vi "OutputDebugString.vi"(6 "Force Log":bool, 8 "error in (log if error)":errorcluster, 11 "log entry string":string) -> (0 "error out":errorcluster, 1 "ms value":u32, 2 "date/time string":string, 3 "data logged":string)   [LabVIEW 2020]
uses:
  Kernel32.dll
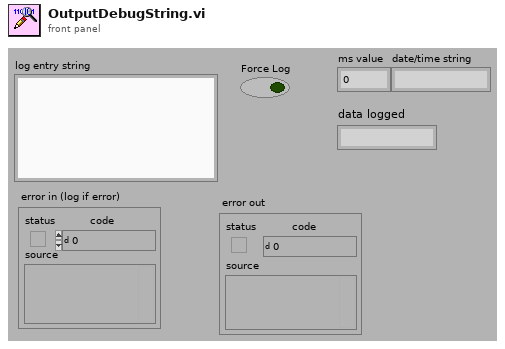
[diagram p1: front panel]
types:
  T1 = enum16{"open", "replace", "create", "open or create", "replace or create", "replace or create with confirmation"}
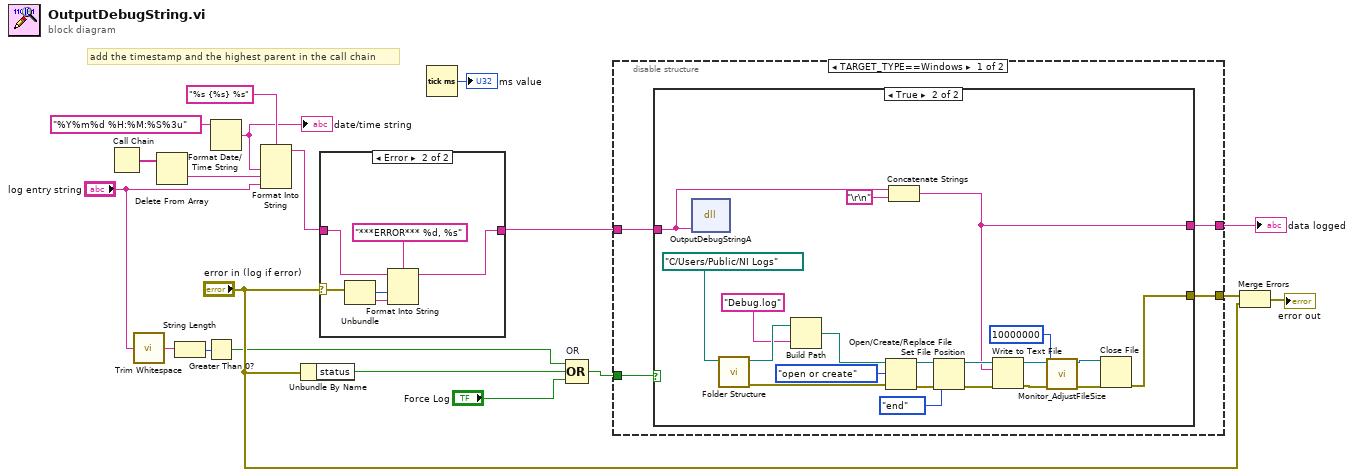
[diagram p0: block diagram]
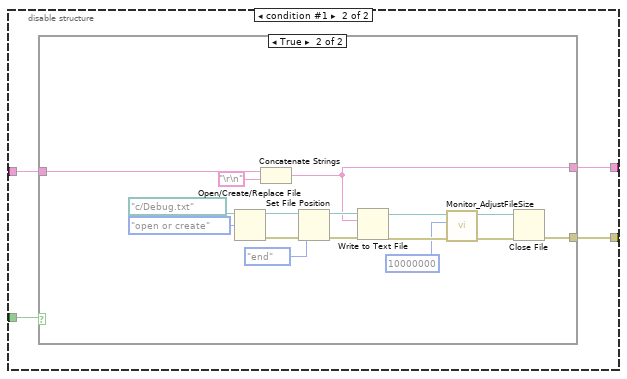
[diagram p3: hidden frame]
diagram:
  # "add the timestamp and the highest parent in the call chain"
  n1 = Call Chain() -> (call chain=w2:string[])
  n2 = call <vilib>:"Trim Whitespace.vi"("string"="log entry string") -> ("trimmed string"=w6:string)  [unwired: 1 in]
  n3 = Delete From Array(array=w2) -> (deleted portion=w1:string)  [unwired: 2 in, 1 out]
  n4 = String Length(string=w6) -> (length=w5:i32)
  n5 = Greater Than 0?(x=w5) -> (x > 0?=w4:bool)
  n6 = Format Date/Time String(time format string (%c)="%Y%m%d %H:%M:%S%3u") -> (date/time string=w9:string)  [unwired: 2 in]
  "date/time string" <- w9
  n7 = Format Into String(format string="%s {%s} %s", w9, w1, "log entry string") -> (resulting string=w8:string)  [unwired: 2 in, 1 out]
  n8 = Unbundle By Name("error in (log if error)") -> ("status"=w18:bool)
  n9 = case shown="Error" "error in (log if error)" {
    selector: "error in (log if error)" -> [_ w25]
    tunnel: w8 -> [w20 w22]
    tunnel: [w20 w21] -> w19
    frame No Error {
    }
    frame Error {
      n10 = Unbundle(w25) -> ("code"=w24:i32, "source"=w23:string)  [unwired: 1 out]
      n11 = Format Into String(format string="***ERROR*** %d, %s", initial string=w22, w24, w23) -> (resulting string=w21:string)  [unwired: 1 in, 1 out]
    }
  }
  n12 = Tick Count (ms)() -> (millisecond timer value=→"ms value":u32)
  n13 = Compound Arithmetic op=OR "OR"(w4, w18, "Force Log") -> (w16:bool)
  n14 = disable-structure shown="TARGET_TYPE==Windows" {
    disable-tunnel: w19 -> [w30 w54]
    disable-tunnel: w16 -> [w29 w53]
    disable-tunnel: [w27 w52] -> w15
    disable-tunnel: [w28 w51] -> w12
    frame condition #0 (active) {
      n15 = case shown="True" w29 {
        tunnel: w30 -> [_ w48]
        tunnel: [_ w37] -> w28
        tunnel: [_ w36] -> w27
        frame False {
        }
        frame True {
          n16 = dll-call lib="kernel32.dll" fn="OutputDebugStringA"("string"=w48) -> ()  [unwired: 5 in, 2 out]
          n17 = call "Folder Structure.vi"("folder structure  to create if nonexistant"=path "C:/Users/Public/NI Logs" ("file path (use dialog)")) -> ("error out"=w31:errorcluster, "directory (dup)"=w34:path)  [unwired: 7 in, 2 out]
          n18 = Build Path(base path=w34, name or relative path="Debug.log") -> (appended path=w33:path)
          n19 = Open/Create/Replace File(file path (use dialog)=w33, error in=w31, operation (0:open)=T1."open or create") -> (refnum out=w44:refnum<file>, error out=w43:errorcluster)  [unwired: 3 in, 1 out]
          n20 = Concatenate Strings(w48, "\r\n") -> (w37:string)
          n21 = Set File Position(refnum=w44, from (0:start)=enum16{"start", "end", "current"}."end", error in=w43) -> (refnum out=w46:refnum<file>, error out=w45:errorcluster)  [unwired: 1 in]
          n22 = Write to Text File(file (use dialog)=w46, text=w37, error in=w45) -> (refnum out=w42:refnum<file>, error out=w41:errorcluster)  [unwired: 1 in, 1 out]
          n23 = call "Monitor_AdjustFileSize.vi"("Error In"=w41, "Max File Size in Bytes"=i64 10000000, "Refnum In"=w42) -> ("Error Out"=w40:errorcluster, "Refnum Out"=w39:refnum<file>)  [unwired: 5 in, 2 out]
          n24 = Close File(refnum=w39, error in=w40) -> (error out=w36:errorcluster)  [unwired: 1 out]
        }
      }
    }
    frame condition #1 {
      n25 = case shown="True" w53 {
        tunnel: w54 -> [_ w63]
        tunnel: [_ w61] -> w52
        tunnel: [_ w55] -> w51
        frame False {
        }
        frame True {
          n26 = Open/Create/Replace File(file path (use dialog)=path "c:/Debug.txt", operation (0:open)=T1."open or create") -> (refnum out=w68:refnum<file>, error out=w66:errorcluster)  [unwired: 4 in, 1 out]
          n27 = Concatenate Strings(w63, "\r\n") -> (w55:string)
          n28 = Set File Position(refnum=w68, from (0:start)=enum16{"start", "end", "current"}."end", error in=w66) -> (refnum out=w65:refnum<file>, error out=w64:errorcluster)  [unwired: 1 in]
          n29 = Write to Text File(file (use dialog)=w65, text=w55, error in=w64) -> (refnum out=w60:refnum<file>, error out=w59:errorcluster)  [unwired: 1 in, 1 out]
          n30 = call "Monitor_AdjustFileSize.vi"("Error In"=w59, "Max File Size in Bytes"=i64 10000000, "Refnum In"=w60) -> ("Error Out"=w57:errorcluster, "Refnum Out"=w58:refnum<file>)  [unwired: 5 in, 2 out]
          n31 = Close File(refnum=w58, error in=w57) -> (error out=w61:errorcluster)  [unwired: 1 out]
        }
      }
    }
  }
  "data logged" <- w12
  n32 = Merge Errors(w15, "error in (log if error)") -> (→"error out":errorcluster)
